vi "Write SelectionMode.vi"(8 "error in (no error)":errorcluster, 10 "SelectionMode":enum16{"CellSelect", "FullRowSelect"}(ring)=enum."FullRowSelect", 11 "DataGridView in":refnum<class "DataGridView.lvclass">) -> (0 "error out":errorcluster, 3 "DataGridView out":refnum<class "DataGridView.lvclass">)   [LabVIEW 2013, in "DataGrid.lvlib" / "DataGridView.lvclass"]
uses:
  DataGridView.lvclass
  System.Windows.Forms
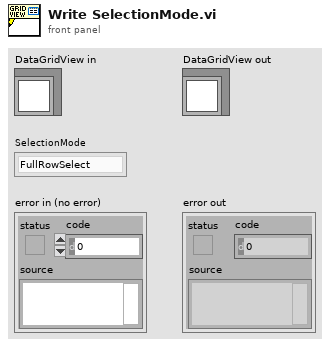
[diagram p1: front panel]
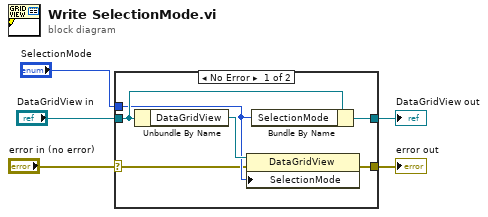
[diagram p0: block diagram]
diagram:
  n1 = case shown="No Error" "error in (no error)" {
    selector: "error in (no error)" -> [w7 w12]
    tunnel: [w6 w12] -> w4
    tunnel: [w11 w13] -> w2
    tunnel: "DataGridView in" -> [w10 w13]
    tunnel: "SelectionMode" -> [w8 _]
    frame No Error {
      n2 = Unbundle By Name(w10) -> ("DataGridView"=w9:refnum<k24>)
      n3 = property class="DataGridView"(reference=w9, error in=w7, "SelectionMode"=w8) -> (error out=w6:errorcluster)  [unwired: 1 out]
      n4 = Bundle By Name(cluster=w10, "SelectionMode"=w8) -> (w11:refnum<class "DataGridView.lvclass">)
    }
    frame Error {
    }
  }
  "error out" <- w4
  "DataGridView out" <- w2
